vi "Different.vi"() -> ()   [LabVIEW 2017, in "Assertions.Tests.lvlib" / "Assert Not Equals.lvlib"]
uses:
  Assert Not Equals.lvlib
  1f9a11cc-cfa7-4d0b-86bd-96debd215748.vi
  src/Transparent Assertions/Constraints/IsEqual/IsEqual.lvclass
  C:/Users/pasca/Projects/Home/TransparentAssertions/src/Transparent Assertions/Constraints/Constraint/Constraint.lvclass
  src/Transparent Assertions/Constraints/IsEqual/Create.vi
  src/Transparent Assertions/Constraints/LogicalNot/LogicalNot.lvclass
  src/Transparent Assertions/Constraints/UnaryOperator/UnaryOperator.lvclass
  src/Transparent Assertions/Assertions/Assertions.lvlib
panel:
  out "error out":errorcluster
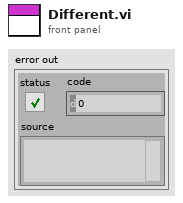
[diagram p1: front panel]
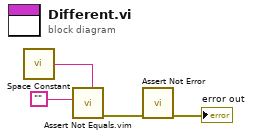
[diagram p0: block diagram]
diagram:
  n1 = call <vilib>:"Space Constant.vi"() -> ("String"=w3:string)
  n2 = call "Assert Not Equals.vim"("Expected"=w3, "Actual"="") -> ("error out"=w2:errorcluster)  [unwired: 9 in]
  n3 = call "Assert Not Error.vi"("error in (no error)"=w2) -> ("error out"=→"error out":errorcluster)  [unwired: 10 in]
